vi "Initialize.vi"(8 "error in (no error)":errorcluster, 11 "VISA resource name":refnum<visa-resource-name>="COM1") -> (0 "error out":errorcluster, 3 "VISA resource name out":refnum<visa-resource-name>)   [LabVIEW 2009, in "Digikrom DK24x.lvlib"]
doc: "Initializes the serial port and returns a new VISA session."
uses:
  Digikrom DK24x.lvlib
  <vilib>/Instr/_visa.llb/VISA Configure Serial Port (Instr).vi
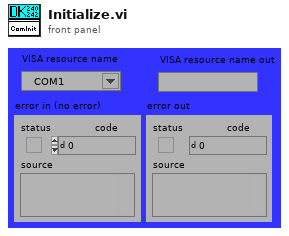
[diagram p1: front panel]
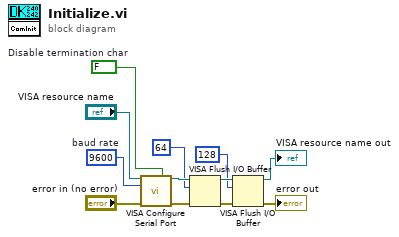
[diagram p0: block diagram]
diagram:
  w11 = u16 9600  # baud rate
  w2 = FALSE  # Disable termination char
  n1 = call-poly "VISA Configure Serial Port"("VISA resource name"="VISA resource name", "Enable Termination\nChar (T)"=w2, "baud rate (9600)"=w11, "error in (no error)"="error in (no error)") -> ("VISA resource name out"=w6:refnum<visa-resource-name>, "error out"=w7:errorcluster)  [unwired: 3 in, 7 out]
  n2 = VISA Flush I/O Buffer(VISA resource name=w6, mask (16)=64, error in (no error)=w7) -> (VISA resource name out=w5:refnum<visa-resource-name>, error out=w8:errorcluster)
  n3 = VISA Flush I/O Buffer(VISA resource name=w5, mask (16)=128, error in (no error)=w8) -> (VISA resource name out=→"VISA resource name out":refnum<visa-resource-name>, error out=→"error out":errorcluster)
